vi "PI_simpl_gain_sched.vi"(6 "KI_derate":sgl format="%#_13g", 8 "ze_sched_thresh":sgl, 9 "ze":sgl, 10 "raster-scan-params":T1={"TsTicks"=1600, "Stop"=FALSE, "TOL"=0.3, "ramp-rate"=0.0, "z-u-max"=5.0, "PI-params"={"Ki"=0.0, "setpoint"=0.0}, "Num"=[-0.00254, 0.000408, 0.00295, 0.0, 0.0, 0.0, 0.0, 0.0, 0.0], "TF Order"=2, "Den"=[0.982758, -1.98194, 1.0, 0.0, 0.0, 0.0, 0.0, 0.0, 0.0]} {"ramp-rate" format="%#_13g"; "TOL" format="%#_13g"}, 11 "u(k-1)":sgl format="%#_13g") -> (2 "u(k)":sgl)   [LabVIEW 2017]
uses:
  raster-scan-params.ctl
  controls/PI-params.ctl
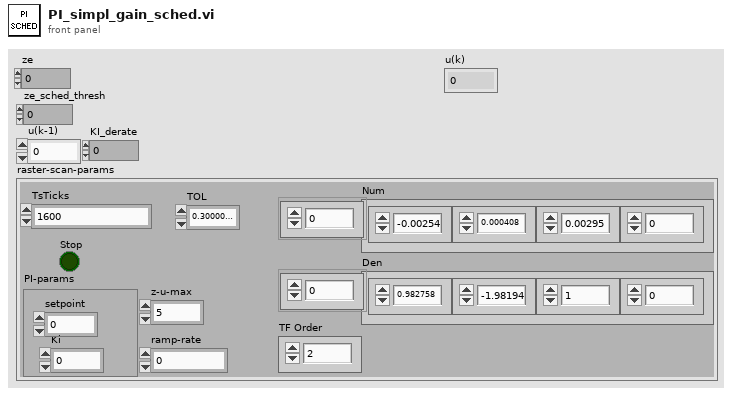
[diagram p1: front panel]
types:
  T1 = typedef "raster-scan-params.ctl" = cluster{"TsTicks":u32, "Stop":bool, "TOL":sgl, "ramp-rate":sgl, "z-u-max":sgl, "PI-params":T2, "Num":sgl[], "TF Order":i32, "Den":sgl[]}
  T2 = typedef "PI-params.ctl" = cluster{"Ki":sgl, "setpoint":sgl}
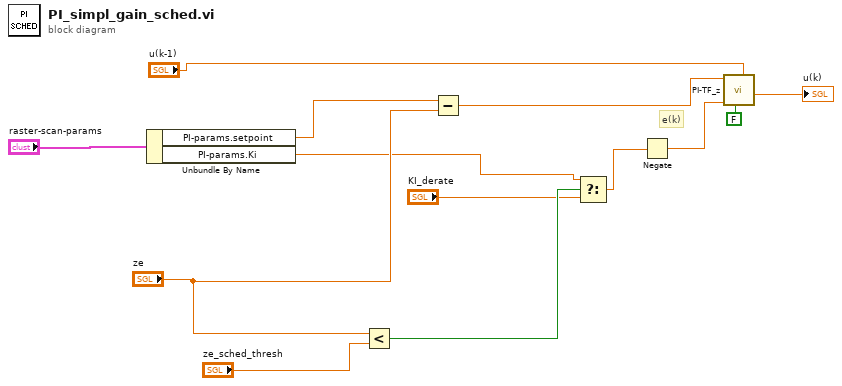
[diagram p0: block diagram]
diagram:
  # "e(k)"
  n1 = Unbundle By Name("raster-scan-params") -> ("PI-params.setpoint"=w13:sgl, "PI-params.Ki"=w3:sgl)
  n2 = Less?(x="ze", y="ze_sched_thresh") -> (x < y?=w4:bool)
  n3 = Subtract(x=w13, y="ze") -> (x-y=w11:sgl)
  n4 = Select(t=w3, s=w4, f="KI_derate") -> (s? t:f=w9:sgl)
  n5 = Negate(x=w9) -> (-x=w10:sgl)
  n6 = call "PI-TF_z.vi"("u(k-1)"="u(k-1)", "reset"=FALSE, "Ki"=w10, "e(k)"=w11) -> ("u(k)"=→"u(k)":sgl)  [unwired: 7 in]
